vi "Close.vi"(8 "error in (no error)":errorcluster, 11 "Rename in":refnum<class "ProjectItem.lvclass">) -> (0 "error out":errorcluster, 3 "Rename out":refnum<class "ProjectItem.lvclass">)   [LabVIEW 2019, in "ProjectItem.lvclass"]
uses:
  ProjectItem.lvclass
  ProjectItem.lvclass/ProjectItem.ctl
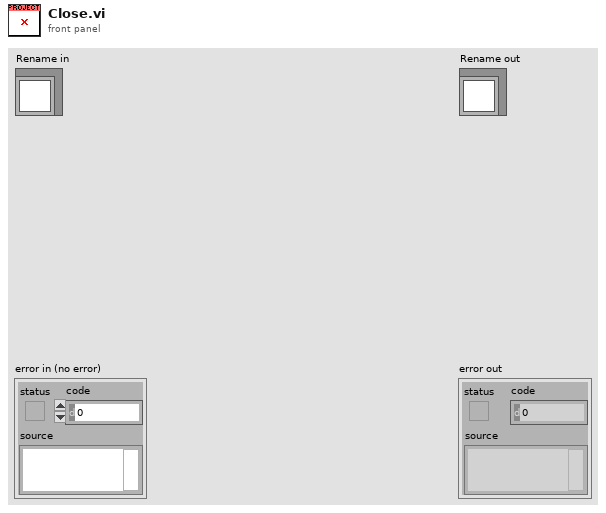
[diagram p1: front panel]
types:
  T1 = cluster{"Class":refnum<vi>, "DynamicVIs":refnum<vi>[], "StaticVIs":refnum<vi>[]}[]
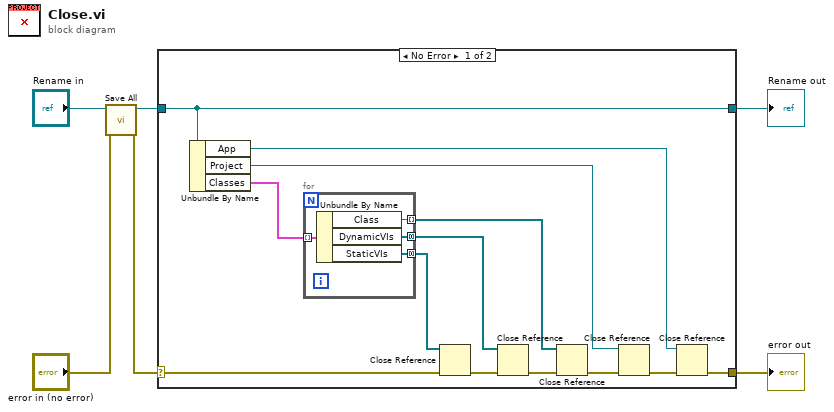
[diagram p0: block diagram]
diagram:
  n1 = call "Save All.vi"("error in (no error)"="error in (no error)", "Rename in"="Rename in") -> ("error out"=w1:errorcluster, "Rename out"=w3:refnum<class "ProjectItem.lvclass">)  [unwired: 8 in]
  n2 = case shown="No Error" w1 {
    selector: w1 -> [w12 w25]
    tunnel: [w19 w25] -> w6
    tunnel: [w8 w24] -> w5
    tunnel: w3 -> [w8 w24]
    frame No Error {
      n3 = Unbundle By Name(w8) -> ("App"=w10:refnum<vi>, "Project"=w9:refnum<vi>, "Classes"=w7:T1)
      n4 = for {
        tunnel: w7 -> [w23] mode=indexing
        tunnel: [w22] -> w16 mode=concatenating
        tunnel: [w21] -> w13 mode=concatenating
        tunnel: [w20] -> w14 mode=indexing
        n5 = Unbundle By Name(w23) -> ("Class"=w20:refnum<vi>, "DynamicVIs"=w21:refnum<vi>[], "StaticVIs"=w22:refnum<vi>[])
      }
      n6 = Close Reference(reference=w16, error in (no error)=w12) -> (error out=w18:errorcluster)
      n7 = Close Reference(reference=w13, error in (no error)=w18) -> (error out=w15:errorcluster)
      n8 = Close Reference(reference=w14, error in (no error)=w15) -> (error out=w11:errorcluster)
      n9 = Close Reference(reference=w9, error in (no error)=w11) -> (error out=w17:errorcluster)
      n10 = Close Reference(reference=w10, error in (no error)=w17) -> (error out=w19:errorcluster)
    }
    frame Error {
    }
  }
  "error out" <- w6
  "Rename out" <- w5
